vi "reinitializeController.vi"(8 "error in (no error)":errorcluster, 11 "Model in":refnum<class "Model.lvclass">) -> (0 "error out":errorcluster, 3 "Model out":refnum<class "Model.lvclass">)   [LabVIEW 2013, in "Model.lvclass"]
uses:
  Model.lvclass
  Model.lvclass/Model.ctl
  ApplicationElements/SystemController/SystemController.lvclass/SystemController.ctl
  ApplicationElements/SystemController/SystemController.lvclass
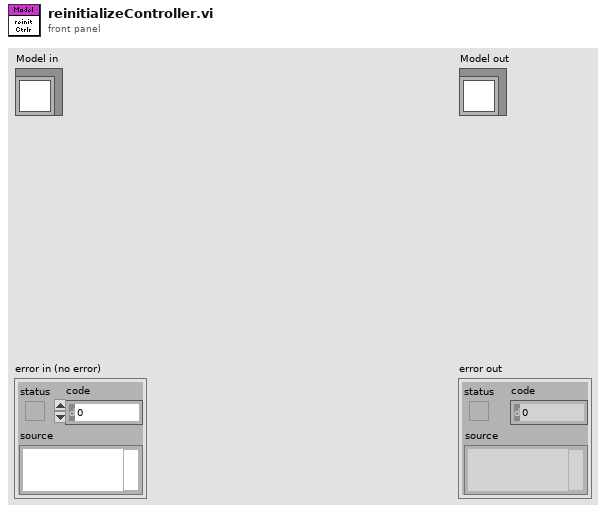
[diagram p1: front panel]
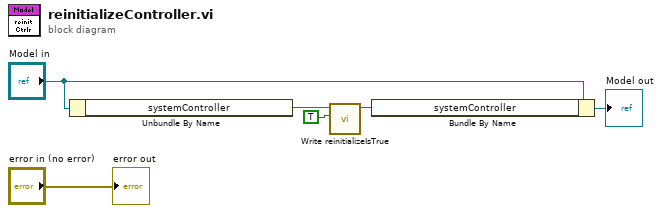
[diagram p0: block diagram]
diagram:
  n1 = Unbundle By Name("Model in") -> ("systemController"=w5:refnum<class "SystemController.lvclass">)
  n2 = call "Write reinitializeIsTrue.vi"("reinitializeIsTrue"=TRUE, "SystemController in"=w5) -> ("SystemController out"=w4:refnum<class "SystemController.lvclass">)  [unwired: 9 in]
  n3 = Bundle By Name(cluster="Model in", "systemController"=w4) -> (→"Model out":refnum<class "Model.lvclass">)
  "error out" <- "error in (no error)"
